vi "Connection Mode Generation Connections List_Initialize.vi"(8 "error in (no error)":errorcluster) -> (0 "error out":errorcluster {"code" min=0 max=0}, 3 "CM Gen Ref out":T1)   [LabVIEW 2013, in "J1939.lvlib"]
uses:
  J1939.lvlib
  Connection Mode Generation Connection Ref.ctl
  TP/TP Connections List State.ctl
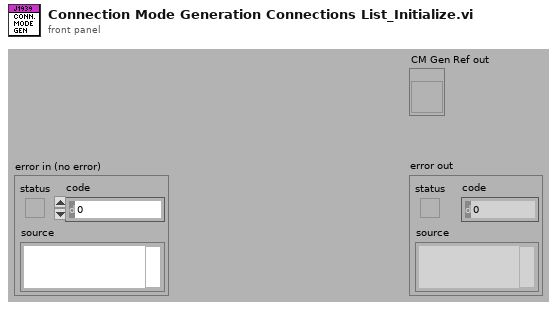
[diagram p1: front panel]
types:
  T1 = typedef "J1939.lvlib/Connection Mode Generation Connection Ref.ctl" = refnum<vi>
  T2 = typedef "J1939.lvlib/TP Connections List State.ctl" = enum16{"Add", "Update", "Get", "Remove", "Initialize"}
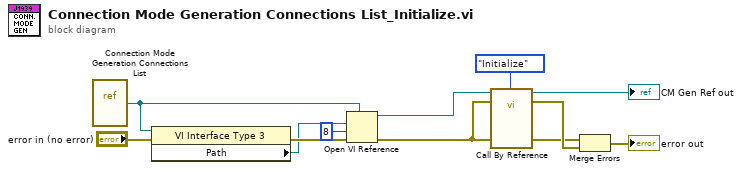
[diagram p0: block diagram]
diagram:
  n1 = vi-ref "Connection Mode Generation Connections List.vi"() -> (w12:refnum<vi>)
  n2 = property class="VI Interface Type 3"(reference=w12, error in="error in (no error)") -> (error out=w10:errorcluster, "Path"=w7:path)  [unwired: 1 out]
  n3 = Open VI Reference(type specifier VI Refnum (for type only)=w12, vi path=w7, options=8, error in (no error)=w10) -> (vi reference=w6:refnum<vi>, error out=w4:errorcluster)  [unwired: 2 in]
  n4 = call-by-ref "?"(reference=w6, error in=w4, "State"=TP_Connections_List_State."Initialize", 11:"error in (no error)"=w4) -> (reference out=→"CM Gen Ref out":refnum<vi>, error out=w5:errorcluster, 15:"error out"=w3:errorcluster)  [unwired: 11 in, 2 out]
  n5 = Merge Errors(w3, w5) -> (→"error out":errorcluster)
